vi "StateActionAnalyser.vi"(1 "FoundObjectOnWire":T3, 7 "CaseStatesIn(IgnoredIfNotWired)":string[](array[string]), 9 "StateActionIn(IgnoredIfNotWired)":T1[](array[typedef])) -> (15 "CaseState":string, 16 "StateAction":T1={"State(s)"="", "StateAction"=enum."AddIfNothingInQueue", "Arg(s)"="", "Comment(s)"=""}, 17 "Linked to the Parse State Queue VI":bool)   [LabVIEW 2014, in "StateReverse.lvclass"]
uses:
  <resource>/Framework/Providers/Open_GDS/UML/StateReverse_class/StateReverse.lvclass
  <resource>/Framework/Providers/Open_GDS/UML/StateReverse_class/NextStateAction.ctl
  <resource>/Framework/Providers/Open_GDS/UML/StateReverse_class/StateAction.ctl
  <resource>/Framework/Providers/Open_GDS/ClassProviders/Common/ScriptingFunctions/Scripting_PastThroughObjectType.ctl
  <resource>/Framework/Providers/Open_GDS/ClassProviders/Common/ScriptingFunctions/Scripting_ObjectType.ctl
  <resource>/Framework/Providers/Open_GDS/ClassProviders/Common/ScriptingFunctions/Scripting.lvclass
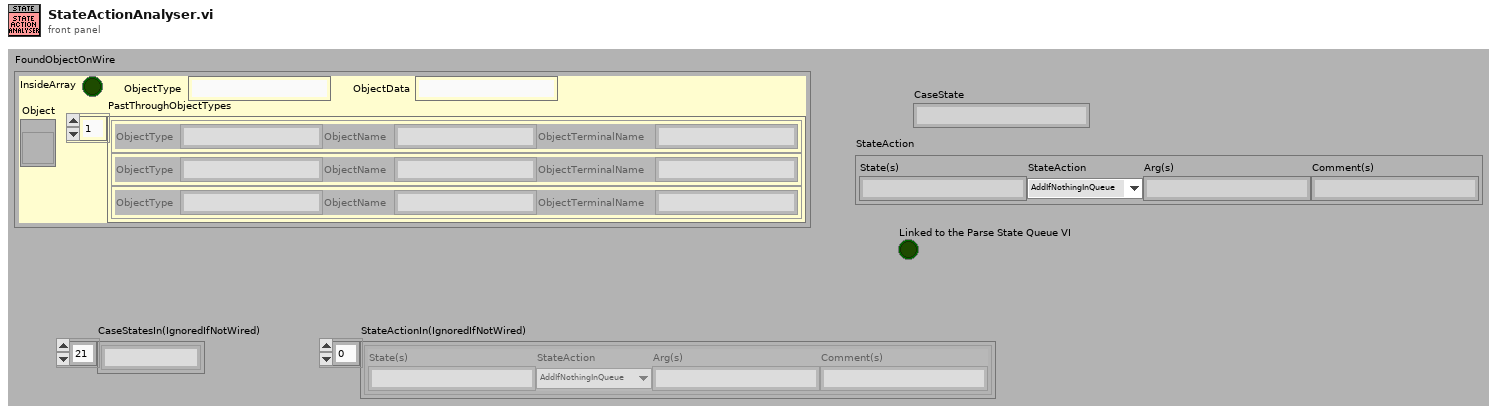
[diagram p1: front panel]
types:
  T1 = typedef "StateReverse.lvclass/NextStateAction.ctl" = cluster{"State(s)":string, "StateAction":T2, "Arg(s)":string, "Comment(s)":string}
  T2 = typedef "StateReverse.lvclass/StateAction.ctl" = enum16{"Normal", "AddInBeggining", "AddInEnd", "AddIfNothingInQueue"}
  T3 = typedef "Scripting.lvclass/Scripting_PastThroughObjectType.ctl" = cluster{"Object":refnum<vi>, "InsideArray":bool, "PastThroughObjectTypes":T4[], "ObjectType":string, "ObjectData":string}
  T4 = typedef "Scripting_ObjectType.ctl" = cluster{"ObjectType":string, "ObjectName":string, "ObjectTerminalName":string}
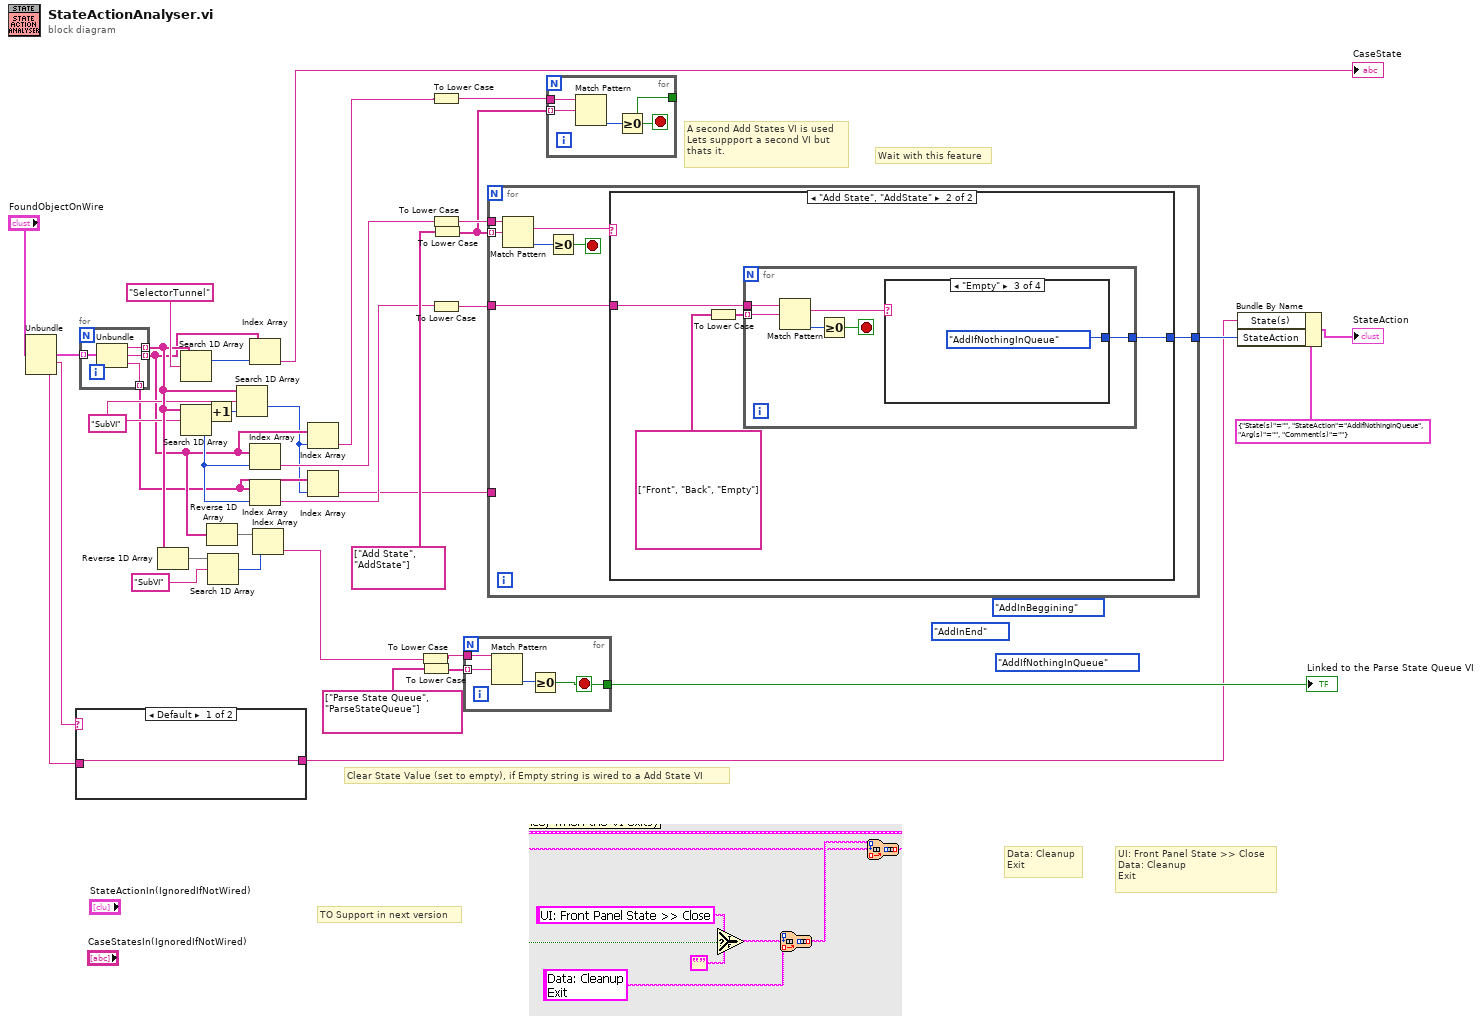
[diagram p0: block diagram]
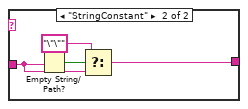
[diagram p2: hidden frame]
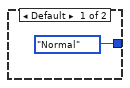
[diagram p3: hidden frame]
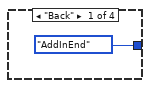
[diagram p4: hidden frame]
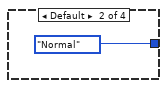
[diagram p5: hidden frame]
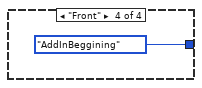
[diagram p6: hidden frame]
diagram:
  w11 = "SubVI" ("x")
  (unwired) StateAction."AddIfNothingInQueue" ("StateAction")
  (unwired) StateAction."AddInEnd" ("StateAction")
  (unwired) StateAction."AddInBeggining" ("StateAction")
  # "Wait with this feature"
  # "TO Support in next version"
  # "UI: Front Panel State >> Close\nData: Cleanup\nExit"
  # "Data: Cleanup\nExit"
  # "A second Add States VI is used\nLets suppport a second VI but\nthats it."
  # "Clear State Value (set to empty), if Empty string is wired to a Add State VI"
  n1 = Unbundle("FoundObjectOnWire") -> ("PastThroughObjectTypes"=w34:T4[], "ObjectType"=w3:string, "ObjectData"=w2:string)  [unwired: 2 out]
  n2 = case shown="Default" w3 {
    tunnel: w2 -> [w37 w40]
    tunnel: [w37 w38] -> w1
    frame Default {
    }
    frame "StringConstant" {
      n3 = Empty String/Path?(string/path=w40) -> (empty?=w41:bool)
      n4 = Select(t="\"\"", s=w41, f=w40) -> (s? t:f=w38:string)
    }
  }
  n5 = for {
    tunnel: w34 -> [w45] mode=indexing
    tunnel: [w44] -> w10 mode=indexing
    tunnel: [w43] -> w9 mode=indexing
    tunnel: [w42] -> w12 mode=indexing
    n6 = Unbundle(w45) -> ("ObjectType"=w42:string, "ObjectName"=w44:string, "ObjectTerminalName"=w43:string)
  }
  n7 = Reverse 1D Array(array=w12) -> (reversed array=w21:string[])
  n8 = Search 1D Array(1D array=w12, element="SelectorTunnel" ("x")) -> (index of element=w32:i32)  [unwired: 1 in]
  n9 = Search 1D Array(1D array=w12, element=w11) -> (index of element=w13:i32)  [unwired: 1 in]
  n10 = Increment(x=w13) -> (x+1=w7:i32)
  n11 = Reverse 1D Array(array=w10) -> (reversed array=w19:string[])
  n12 = Search 1D Array(1D array=w21, element="SubVI" ("x")) -> (index of element=w18:i32)  [unwired: 1 in]
  n13 = Search 1D Array(1D array=w12, element=w11, start index (0)=w7) -> (index of element=w8:i32)
  n14 = Index Array(array=w10, index=w32) -> (element=→"CaseState":string)
  n15 = Index Array(array=w10, index=w13) -> (element=w17:string)
  n16 = Index Array(array=w9, index=w13) -> (element=w27:string)
  n17 = Index Array(array=w19, index=w18) -> (element=w16:string)
  n18 = Index Array(array=w10, index=w8) -> (element=w6:string)
  n19 = Index Array(array=w9, index=w8) -> (element=w4:string)
  n20 = To Lower Case(string=w16) -> (all lower case string=w25:string)
  n21 = To Lower Case(string=string[] ["Parse State Queue", "ParseStateQueue"]) -> (all lower case string=w23:string[])
  n22 = To Lower Case(string=w6) -> (all lower case string=w5:string)
  n23 = To Lower Case(string=w17) -> (all lower case string=w15:string)
  n24 = To Lower Case(string=w27) -> (all lower case string=w35:string)
  n25 = To Lower Case(string=string[] ["Add State", "AddState"]) -> (all lower case string=w14:string[])
  n26 = for {
    tunnel: w25 -> [w49]
    tunnel: w23 -> [w48] mode=indexing
    tunnel: [w46] -> w22
    stop <- w46 stop-if-true
    n27 = Match Pattern(string=w49, regular expression=w48) -> (offset past match=w47:i32)  [unwired: 1 in, 3 out]
    n28 = Greater Or Equal To 0?(x=w47) -> (x >= 0?=w46:bool)
  }
  "Linked to the Parse State Queue VI" <- w22
  n29 = for {
    tunnel: w15 -> [w56]
    tunnel: w14 -> [w55] mode=indexing
    tunnel: w35 -> [w53]
    tunnel: [w51] -> w29
    tunnel: w4 -> [_]
    stop <- w54 stop-if-true
    n30 = Match Pattern(string=w56, regular expression=w55) -> (match substring=w52:string, offset past match=w50:i32)  [unwired: 1 in, 2 out]
    n31 = Greater Or Equal To 0?(x=w50) -> (x >= 0?=w54:bool)
    n32 = case shown="\"Add State\", \"AddState\"" w52 {
      tunnel: w53 -> [_ w61]
      tunnel: [StateAction."Normal" ("StateAction") w58] -> w51
      frame Default {
      }
      frame "Add State", "AddState" {
        n33 = To Lower Case(string=string[] ["Front", "Back", "Empty"]) -> (all lower case string=w59:string[])
        n34 = for {
          tunnel: w61 -> [w67]
          tunnel: w59 -> [w64] mode=indexing
          tunnel: [w62] -> w58
          stop <- w65 stop-if-true
          n35 = Match Pattern(string=w67, regular expression=w64) -> (match substring=w63:string, offset past match=w66:i32)  [unwired: 1 in, 2 out]
          n36 = Greater Or Equal To 0?(x=w66) -> (x >= 0?=w65:bool)
          n37 = case shown="\"Empty\"" w63 {
            tunnel: [StateAction."AddInEnd" ("StateAction") StateAction."Normal" ("StateAction") StateAction."AddIfNothingInQueue" ("StateAction") StateAction."AddInBeggining" ("StateAction")] -> w62
            frame "Back" {
            }
            frame Default {
            }
            frame "Empty" {
            }
            frame "Front" {
            }
          }
        }
      }
    }
  }
  n38 = for {
    tunnel: w5 -> [w75]
    tunnel: w14 -> [w74] mode=indexing
    tunnel: [w72] -> _
    stop <- w72 stop-if-true
    n39 = Match Pattern(string=w75, regular expression=w74) -> (offset past match=w73:i32)  [unwired: 1 in, 3 out]
    n40 = Greater Or Equal To 0?(x=w73) -> (x >= 0?=w72:bool)
  }
  n41 = Bundle By Name(cluster=T1 {"State(s)"="", "StateAction"=enum."AddIfNothingInQueue", "Arg(s)"="", "Comment(s)"=""} ("StateAction"), "State(s)"=w1, "StateAction"=w29) -> (→"StateAction":T1)
